vi "Calculate Angles Motors.vi"(6 "Prev Flip Speeds?":bool[](array[boolean]), 7 "PID gains":T1={"proportional gain (Kc)"=0.02, "integral time (Ti, min)"=0.0, "derivative time (Td, min)"=0.0} {"proportional gain (Kc)" format="%_6f"; "integral time (Ti, min)" format="%_6f"; "derivative time (Td, min)" format="%_6f"}, 8 "Speeds":dbl[](array[numeric]), 11 "Angles":dbl[](array[numeric])) -> (0 "Flip Speeds?":bool[](array[boolean]), 3 "Angle Motor Outputs":dbl[](array[numeric]))   [LabVIEW 2020]
uses:
  <vilib>/Rock Robotics/Network Tables/NT Write Numeric Array.vi
  <vilib>/addons/control/pid/pid.llb/PID (DBL).vi
  <vilib>/addons/control/pid/NI_PID_pid.lvlib
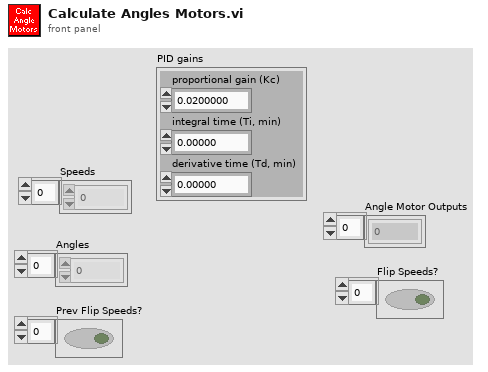
[diagram p1: front panel]
types:
  T1 = cluster{"proportional gain (Kc)":dbl, "integral time (Ti, min)":dbl, "derivative time (Td, min)":dbl}
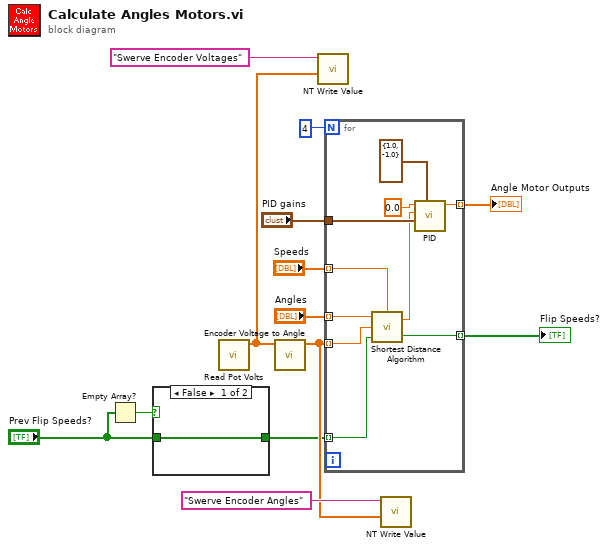
[diagram p0: block diagram]
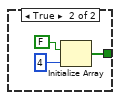
[diagram p2: hidden frame]
diagram:
  n1 = Empty Array?(array="Prev Flip Speeds?") -> (empty?=w5:bool)
  n2 = case shown="False" w5 {
    tunnel: [w14 w17] -> w4
    tunnel: "Prev Flip Speeds?" -> [w14 _]
    frame False {
    }
    frame True {
      n3 = Initialize Array(FALSE, 4 ("dimension size")) -> (w17:bool[])
    }
  }
  n4 = call "Read Pot Volts.vi"() -> ("Encoder Voltages"=w1:dbl[])  [unwired: 11 in]
  n5 = call "Encoder Voltage to Angle.vi"("Encoder Voltages"=w1) -> ("Angle"=w9:dbl[])  [unwired: 10 in]
  n6 = call-poly <vilib>:"NT Write Value.vi"("Numeric Array"=w1, "Name"="Swerve Encoder Voltages") -> ()  [unwired: 9 in, 1 out]
  n7 = for {
    N: 4 -> [_]
    tunnel: "PID gains" -> [w27]
    tunnel: [w24] -> w11 mode=indexing
    tunnel: "Angles" -> [w23] mode=indexing
    tunnel: w9 -> [w22] mode=indexing
    tunnel: [w19] -> w13 mode=indexing
    tunnel: w4 -> [w20] mode=indexing
    tunnel: "Speeds" -> [w18] mode=indexing
    n8 = call "Shortest Distance Algorithm.vi"("Speed"=w18, "Motor Reversed?"=w20, "Encoder Angle"=w22, "Setpoint"=w23) -> ("Reverse Motor"=w19:bool, "PID Input"=w21:dbl)
    n9 = call-poly <vilib>:"PID.vi"("output range"=cluster{"output high":dbl, "output low":dbl} {"output high"=1.0, "output low"=-1.0}, "PID gains"=w27, "process variable"=w21, "setpoint"=0.0) -> ("output"=w24:dbl)  [unwired: 6 in, 1 out]
  }
  "Flip Speeds?" <- w13
  "Angle Motor Outputs" <- w11
  n10 = call-poly <vilib>:"NT Write Value.vi"("Numeric Array"=w9, "Name"="Swerve Encoder Angles") -> ()  [unwired: 9 in, 1 out]
